vi "acc_sensor.vi"() -> ()   [LabVIEW 2018]
uses:
  <vilib>/DAQmx/read.llb/DAQmx Read (Analog 1D DBL NChan 1Samp).vi
  <vilib>/DAQmx/miscellaneous.llb/DAQmx Fill In Error Info.vi
panel:
  out "Waveform Chart 2":cluster{dbl, dbl}[](graph)
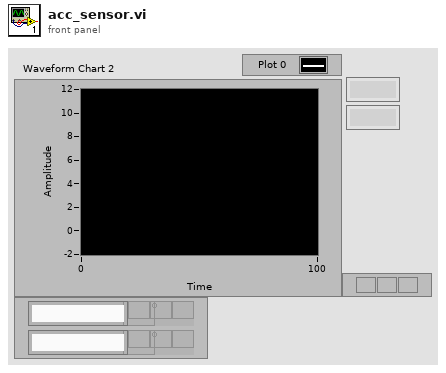
[diagram p1: front panel]
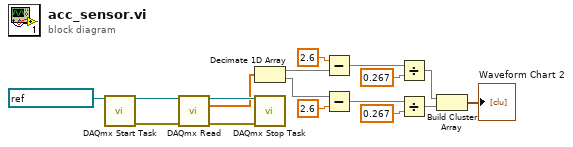
[diagram p0: block diagram]
diagram:
  n1 = call <vilib>:"DAQmx Start Task.vi"("task/channels in"=refnum<k21> "acc_sensor") -> ("task out"=w14:refnum<k21>, "error out"=w16:errorcluster)  [unwired: 13 in]
  n2 = call-poly <vilib>:"DAQmx Read.vi"("task/channels in"=w14, "error in"=w16) -> ("task out"=w15:refnum<k21>, "data"=w12:dbl[], "error out"=w17:errorcluster)  [unwired: 11 in]
  n3 = Decimate 1D Array(w12) -> (w8:dbl[], w7:dbl[])
  n4 = call <vilib>:"DAQmx Stop Task.vi"("task/channels in"=w15, "error in"=w17) -> ()  [unwired: 12 in, 2 out]
  n5 = Subtract(x=2.6, y=w8) -> (x-y=w10:dbl[])
  n6 = Subtract(x=w7, y=2.6) -> (x-y=w5:dbl[])
  n7 = Divide(x=w10, y=0.267) -> (x/y=w3:dbl[])
  n8 = Divide(x=w5, y=0.267) -> (x/y=w2:dbl[])
  n9 = Build Cluster Array(w3, w2) -> (→"Waveform Chart 2":cluster{dbl, dbl}[])
